vi "VI Treevi.vi"   [LabVIEW 2012, in "Phidget BLDC Motor.lvlib"]
doc: "${BLDCMotor:VITreeHeader}"
uses:
  <instrlib>/Phidgets/Phidget BLDC Motor/Phidget BLDC Motor.lvlib
  <instrlib>/Phidgets/Phidget BLDC Motor/Public/BLDCMotorStart.vi
  <instrlib>/Phidgets/Phidget BLDC Motor/Public/BLDCMotorOpen.vi
  <instrlib>/Phidgets/Phidget BLDC Motor/Public/BLDCMotorClose.vi
panel:
  # "(c) 2015 Phidgets Inc..  ALL RIGHTS RESERVED."
  # "SEE DIAGRAM\nFOR VI TREE."
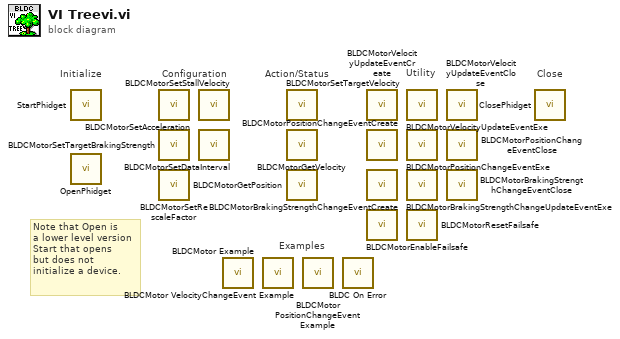
[diagram p0: block diagram]
diagram:
  # "Note that Open is\na lower level version\nStart that opens\nbut does not \ninitialize a device."
  # "Examples"
  # "Configuration"
  # "Utility"
  # "Action/Status"
  # "Close"
  # "Initialize"
  n1 = call-poly <instrlib>:"StartPhidget.vi"() -> ()  [unwired: 12 in, 4 out]
  n2 = call-poly <instrlib>:"OpenPhidget.vi"() -> ()  [unwired: 8 in, 4 out]
  n3 = call <instrlib>:"BLDCMotorSetAcceleration.vi"() -> ()  [unwired: 9 in, 2 out]
  n4 = call <instrlib>:"BLDCMotorSetTargetBrakingStrength.vi"() -> ()  [unwired: 9 in, 2 out]
  n5 = call <instrlib>:"BLDCMotorSetRescaleFactor.vi"() -> ()  [unwired: 9 in, 2 out]
  n6 = call <instrlib>:"BLDCMotorSetStallVelocity.vi"() -> ()  [unwired: 9 in, 2 out]
  n7 = call <instrlib>:"BLDCMotorSetDataInterval.vi"() -> ()  [unwired: 9 in, 2 out]
  n8 = call <instrlib>:"BLDCMotor Example.vi"() -> ()  [unwired: 12 in]
  n9 = call <instrlib>:"BLDCMotor VelocityChangeEvent Example.vi"() -> ()  [unwired: 12 in]
  n10 = call <instrlib>:"BLDCMotorSetTargetVelocity.vi"() -> ()  [unwired: 9 in, 2 out]
  n11 = call <instrlib>:"BLDCMotorGetVelocity.vi"() -> ()  [unwired: 8 in, 3 out]
  n12 = call <instrlib>:"BLDCMotorGetPosition.vi"() -> ()  [unwired: 8 in, 3 out]
  n13 = call <instrlib>:"BLDCMotor PositionChangeEvent Example.vi"() -> ()  [unwired: 12 in]
  n14 = call <instrlib>:"BLDC On Error.vi"() -> ()  [unwired: 12 in]
  n15 = call <instrlib>:"BLDCMotorVelocityUpdateEventCreate.vi"() -> ()  [unwired: 9 in, 3 out]
  n16 = call <instrlib>:"BLDCMotorPositionChangeEventCreate.vi"() -> ()  [unwired: 9 in, 3 out]
  n17 = call <instrlib>:"BLDCMotorBrakingStrengthChangeEventCreate.vi"() -> ()  [unwired: 9 in, 3 out]
  n18 = call <instrlib>:"BLDCMotorEnableFailsafe.vi"() -> ()  [unwired: 9 in, 2 out]
  n19 = call <instrlib>:"BLDCMotorVelocityUpdateEventExe.vi"() -> ()  [unwired: 5 in, 7 out]
  n20 = call <instrlib>:"BLDCMotorPositionChangeEventExe.vi"() -> ()  [unwired: 5 in, 7 out]
  n21 = call <instrlib>:"BLDCMotorBrakingStrengthChangeUpdateEventExe.vi"() -> ()  [unwired: 5 in, 7 out]
  n22 = call <instrlib>:"BLDCMotorResetFailsafe.vi"() -> ()  [unwired: 9 in, 2 out]
  n23 = call <instrlib>:"BLDCMotorVelocityUpdateEventClose.vi"() -> ()  [unwired: 10 in, 2 out]
  n24 = call <instrlib>:"BLDCMotorPositionChangeEventClose.vi"() -> ()  [unwired: 10 in, 2 out]
  n25 = call <instrlib>:"BLDCMotorBrakingStrengthChangeEventClose.vi"() -> ()  [unwired: 10 in, 2 out]
  n26 = call-poly <instrlib>:"ClosePhidget.vi"() -> ()  [unwired: 11 in, 1 out]
